vi "Handle Error.vi"(8 "error in (no error)":errorcluster, 11 "DAQ_Module in":refnum<class "DAQ_Module.lvclass">) -> (0 "error out":errorcluster, 2 "stop actor?":bool=TRUE, 3 "DAQ_Module out":refnum<class "DAQ_Module.lvclass">)   [LabVIEW 2025, in "DAQ_Module.lvlib" / "DAQ_Module.lvclass"]
doc: "<p>(<strong>Filename</strong>: <span class=\"dnl\">Actor Framework.lvlib:Actor.lvclass:Handle Error.vi</span>)</p>\n<p>Defines how the actor handles an error that occurred while processing a message. By default, this method does nothing except stop the actor.</p>"
uses:
  DAQ_Module.lvclass
  Module/Module/Module/Module.lvclass
  DAQ_Module.lvclass/DAQ_Module.ctl
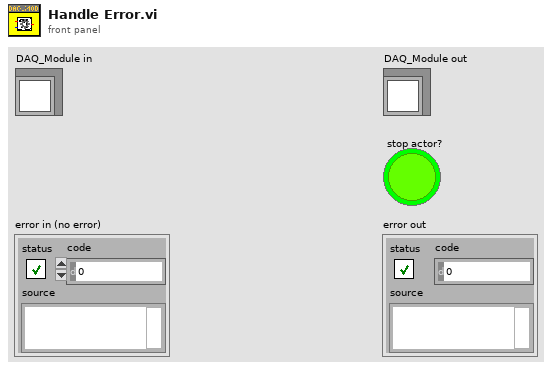
[diagram p1: front panel]
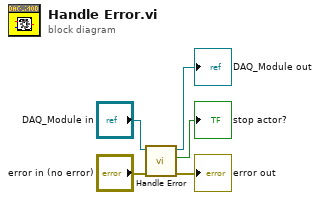
[diagram p0: block diagram]
diagram:
  n1 = call-parent "Handle Error.vi"("error in (no error)"="error in (no error)", "Actor in"="DAQ_Module in") -> ("error out"=→"error out":errorcluster, "stop actor?"=→"stop actor?":bool, "Actor out"=→"DAQ_Module out":refnum<class "DAQ_Module.lvclass">)  [unwired: 7 in]
